vi "SDKSID4_Get User Profile.vi"(0 "SDKSID4 session In":T4, 7 "error in":errorcluster) -> (10 "SDK Version":string, 12 "UserProfileName":string, 14 "UserProfile_File":string, 16 "UserProfileDescription":string, 18 "UserProfile_LastReference":string, 20 "SDKSID4 session Out":T4, 21 "UserProfileDirectory":string, 22 "SNPhasics":string, 23 "Analysis info":T2, 24 "Camera info":T3, 25 "ImageCameraSize":T1, 27 "error out":errorcluster)   [LabVIEW 2013]
doc: "This function outputs the parameters currently used. Three clusters (or structs in C) are given. One describes the interferogram analysis parameters (<B>Analysis Info</B>). The other one enumerates the current camera settings (<B>Camera Info</B>). The last one gives information concerning the mirror (<B>OASys Info</B>).\nThese parameters are different from the ones saved in the user profile until you save them using Save Current User Profile."
uses:
  Refnum SDKSID4 session.ctl
  SDKSID4_Camera info.ctl
  SDKSID4_Analysis info.ctl
  SDKSID4_ImageCameraSize.ctl
  SID4_SDK.dll
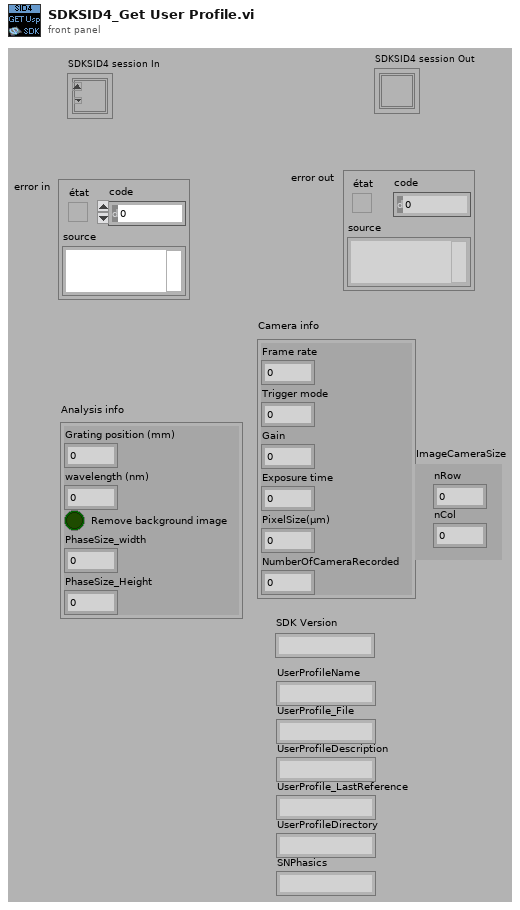
[diagram p1: front panel]
types:
  T1 = typedef "SDKSID4_ImageCameraSize.ctl" = cluster{"nRow":i32, "nCol":i32}
  T2 = typedef "SDKSID4_Analysis info.ctl" = cluster{"Grating position (mm)":dbl, "wavelength (nm)":dbl, "Remove background image":bool, "PhaseSize_width":i32, "PhaseSize_Height":i32}
  T3 = typedef "SDKSID4_Camera info.ctl" = cluster{"Frame rate":i32, "Trigger mode":u32, "Gain":i32, "Exposure time":u32, "PixelSize(µm)":sgl, "NumberOfCameraRecorded":u8}
  T4 = typedef "Refnum SDKSID4 session.ctl" = refnum<k1>
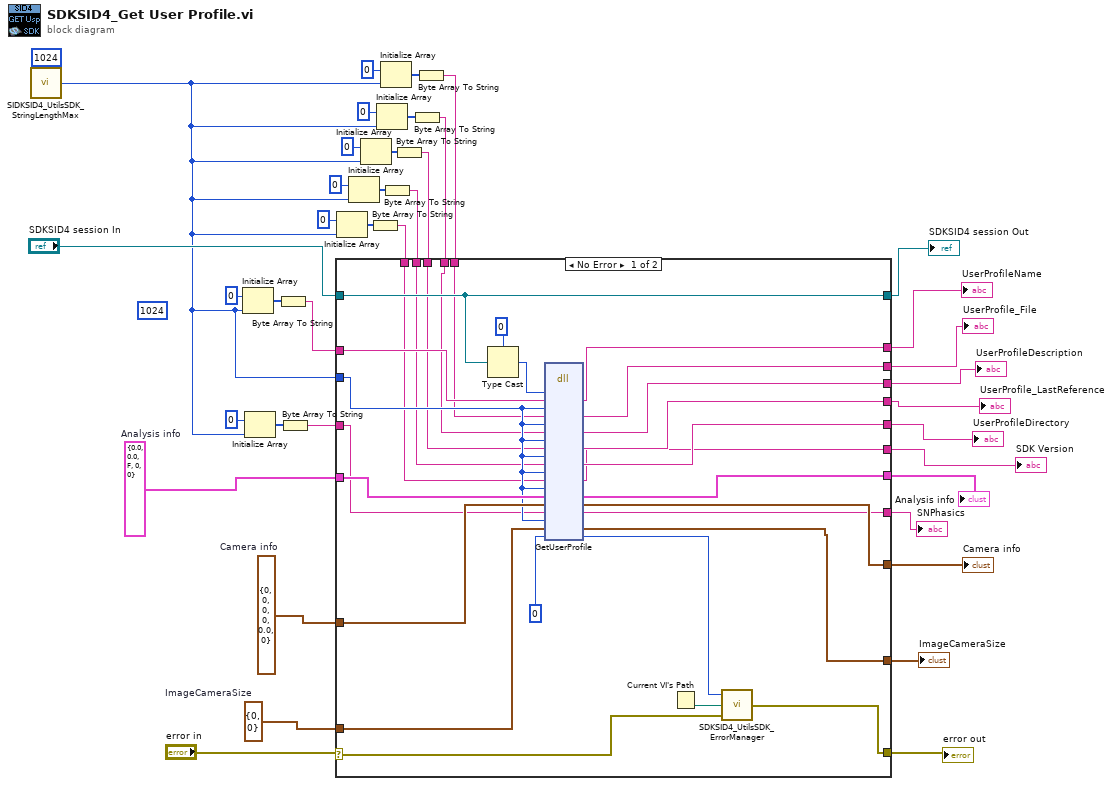
[diagram p0: block diagram]
diagram:
  w3 = T1 {"nRow"=0, "nCol"=0}  # ImageCameraSize
  (unwired) 1024 ("taille de la dimension")
  (unwired) 1024 ("taille de la dimension")
  w35 = T3 {"Frame rate"=0, "Trigger mode"=0, "Gain"=0, "Exposure time"=0, "PixelSize(µm)"=0.0, "NumberOfCameraRecorded"=0}  # Camera info
  w36 = T2 {"Grating position (mm)"=0.0, "wavelength (nm)"=0.0, "Remove background image"=FALSE, "PhaseSize_width"=0, "PhaseSize_Height"=0}  # Analysis info
  n1 = call "SIDKSID4_UtilsSDK_StringLengthMax.vi"() -> ("lgeur max chaine char"=w1:u32)  [unwired: 1 in]
  n2 = Initialize Array(u8 0, w1) -> (w30:u8[])
  n3 = Initialize Array(u8 0, w1) -> (w6:u8[])
  n4 = Byte Array To String(unsigned byte array=w30) -> (string=w29:string)
  n5 = Byte Array To String(unsigned byte array=w6) -> (string=w4:string)
  n6 = Initialize Array(u8 0, w1) -> (w9:u8[])
  n7 = Initialize Array(u8 0, w1) -> (w11:u8[])
  n8 = Initialize Array(u8 0, w1) -> (w15:u8[])
  n9 = Byte Array To String(unsigned byte array=w9) -> (string=w7:string)
  n10 = Initialize Array(u8 0, w1) -> (w17:u8[])
  n11 = Initialize Array(u8 0, w1) -> (w21:u8[])
  n12 = Byte Array To String(unsigned byte array=w11) -> (string=w10:string)
  n13 = Byte Array To String(unsigned byte array=w15) -> (string=w13:string)
  n14 = Byte Array To String(unsigned byte array=w17) -> (string=w16:string)
  n15 = Byte Array To String(unsigned byte array=w21) -> (string=w19:string)
  n16 = case shown="No Error" "error in" {
    selector: "error in" -> [w44 w72]
    tunnel: "SDKSID4 session In" -> [w66 w73]
    tunnel: [w66 w73] -> w39
    tunnel: w36 -> [w62 w71]
    tunnel: w35 -> [w64 w70]
    tunnel: [w45 w72] -> w34
    tunnel: [w61 w71] -> w32
    tunnel: [w63 w70] -> w33
    tunnel: [w65 _] -> w28
    tunnel: w29 -> [w60 _]
    tunnel: w1 -> [w59 _]
    tunnel: [w58 _] -> w27
    tunnel: [w57 _] -> w26
    tunnel: [w56 _] -> w25
    tunnel: [w55 _] -> w24
    tunnel: [w54 _] -> w23
    tunnel: [w53 _] -> w22
    tunnel: w19 -> [w52 _]
    tunnel: w16 -> [w51 _]
    tunnel: w13 -> [w50 _]
    tunnel: w10 -> [w49 _]
    tunnel: w7 -> [w48 _]
    tunnel: w4 -> [w47 _]
    tunnel: w3 -> [w43 w69]
    tunnel: [w42 w69] -> w2
    frame No Error {
      n17 = Type Cast(type=u32 0, x=w66) -> (*(type *) &x=w67:u32)
      n18 = dll-call lib="C:/Program Files/SID4_SDK/DLL SDK/BIN/SID4_SDK.dll" fn="GetUserProfile"("SessionID"=w67, "UserProfileName"=w60, "uspName_bufSize"=w59, "UserProfile_File"=w52, "uspFile_bufSize"=w59, "UserProfileDescription"=w51, "uspDesc_bufSize"=w59, "UserProfile_LastReference"=w50, "uspLastRef_bufSize"=w59, "UserProfileDirectory"=w49, "uspDir_bufSize"=w59, "SDKVersion"=w48, "version__bufSize"=w59, "Analysis info"=w62, "Camera info"=w64, "SNPhasics"=w47, "SNPhasics_bufSize"=w59, "ImageCameraSize"=w43, "ErrorCode"=0) -> ("UserProfileName"=w65:string, "UserProfile_File"=w58:string, "UserProfileDescription"=w57:string, "UserProfile_LastReference"=w56:string, "UserProfileDirectory"=w55:string, "SDKVersion"=w54:string, "Analysis info"=w61:T2, "Camera info"=w63:T3, "SNPhasics"=w53:string, "ImageCameraSize"=w42:T1, "ErrorCode"=w40:i32)  [unwired: 12 in, 2 out]
      n19 = Current VI's Path() -> (path=w46:path)
      n20 = call "SDKSID4_UtilsSDK_ErrorManager.vi"("error IN"=w44, "VI PathFile"=w46, "ErrorCode"=w40) -> ("error OUT"=w45:errorcluster)
    }
    frame Error {
    }
  }
  "error out" <- w34
  "SDKSID4 session Out" <- w39
  "Camera info" <- w33
  "Analysis info" <- w32
  "SDK Version" <- w23
  "UserProfileName" <- w28
  "UserProfile_File" <- w27
  "UserProfileDescription" <- w26
  "UserProfile_LastReference" <- w25
  "UserProfileDirectory" <- w24
  "SNPhasics" <- w22
  "ImageCameraSize" <- w2
